vi "set_constant_intensity.vi"(8 "error in (no error)":errorcluster, 10 "power slider in":cluster{dbl, dbl}, 11 "number of frames":i32) -> (0 "error out":errorcluster, 3 "amplitude out":u16[](array[numeric]))   [LabVIEW 2010, in "TrajectoryMH100122AODRAPS.lvclass"]
uses:
  TrajectoryMH100122AODRAPS.lvclass
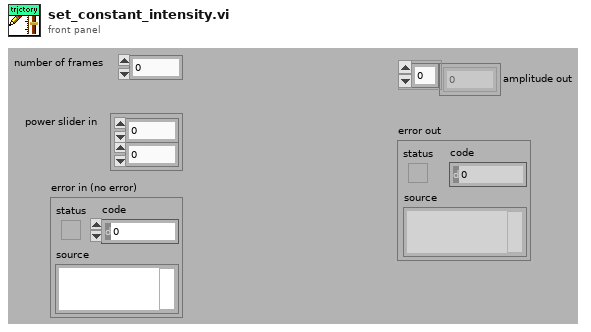
[diagram p1: front panel]
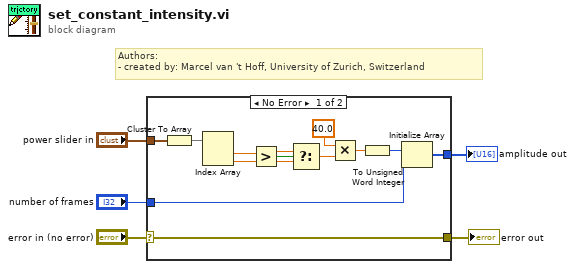
[diagram p0: block diagram]
diagram:
  # "Authors: \n- created by: Marcel van 't Hoff, University of Zurich, Switzerland"
  n1 = case shown="No Error" "error in (no error)" {
    selector: "error in (no error)" -> [w17 w18]
    tunnel: [w17 w18] -> w4
    tunnel: "power slider in" -> [w15 _]
    tunnel: "number of frames" -> [w11 _]
    tunnel: [w10 _] -> w1
    frame No Error {
      n2 = Cluster To Array(cluster=w15) -> (array=w16:dbl[])
      n3 = Index Array(array=w16) -> (element #1=w13:dbl, element #2=w12:dbl)  [unwired: 2 in]
      n4 = Greater?(x=w13, y=w12) -> (0:w14:bool)
      n5 = Select(t=w13, s=w14, f=w12) -> (s? t:f=w7:dbl)
      n6 = Multiply(x=40.0, y=w7) -> (x*y=w6:dbl)
      n7 = To Unsigned Word Integer(number=w6) -> (unsigned 16bit integer=w9:u16)
      n8 = Initialize Array(w9, w11) -> (w10:u16[])
    }
    frame Error {
    }
  }
  "amplitude out" <- w1
  "error out" <- w4
